vi "_PC_RTFunc_MSAnalExeCmd.vi"(5 "sv refnum":T1, 7 "Function":enum16{"Query", "Start", "Pause"}(ring)=enum."Start", 8 "error in (no error)":errorcluster, 9 "MS.Pause":refnum<vi>, 10 "MS.Start":refnum<vi>, 11 "Loops in":i32) -> (0 "error out":errorcluster, 1 "MSAnalExe?":bool, 2 "ExeTimes Out":i32)   [LabVIEW 2018]
uses:
  <vilib>/Utility/error.llb/Error Cluster From Error Code.vi
  <vilib>/ErrorRing/Error Ring.xnode
  <resource>/objmgr/ni.var.rc
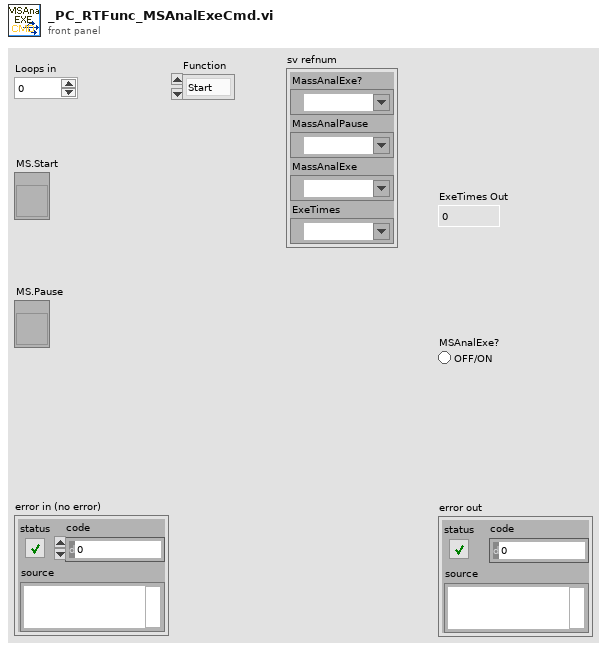
[diagram p1: front panel]
types:
  T1 = cluster{"MassAnalExe?":refnum<k21>, "MassAnalPause":refnum<k21>, "MassAnalExe":refnum<k21>, "ExeTimes":refnum<k21>}
  T2 = enum8{"Enabled", "Disabled", "Disabled and Grayed Out"}
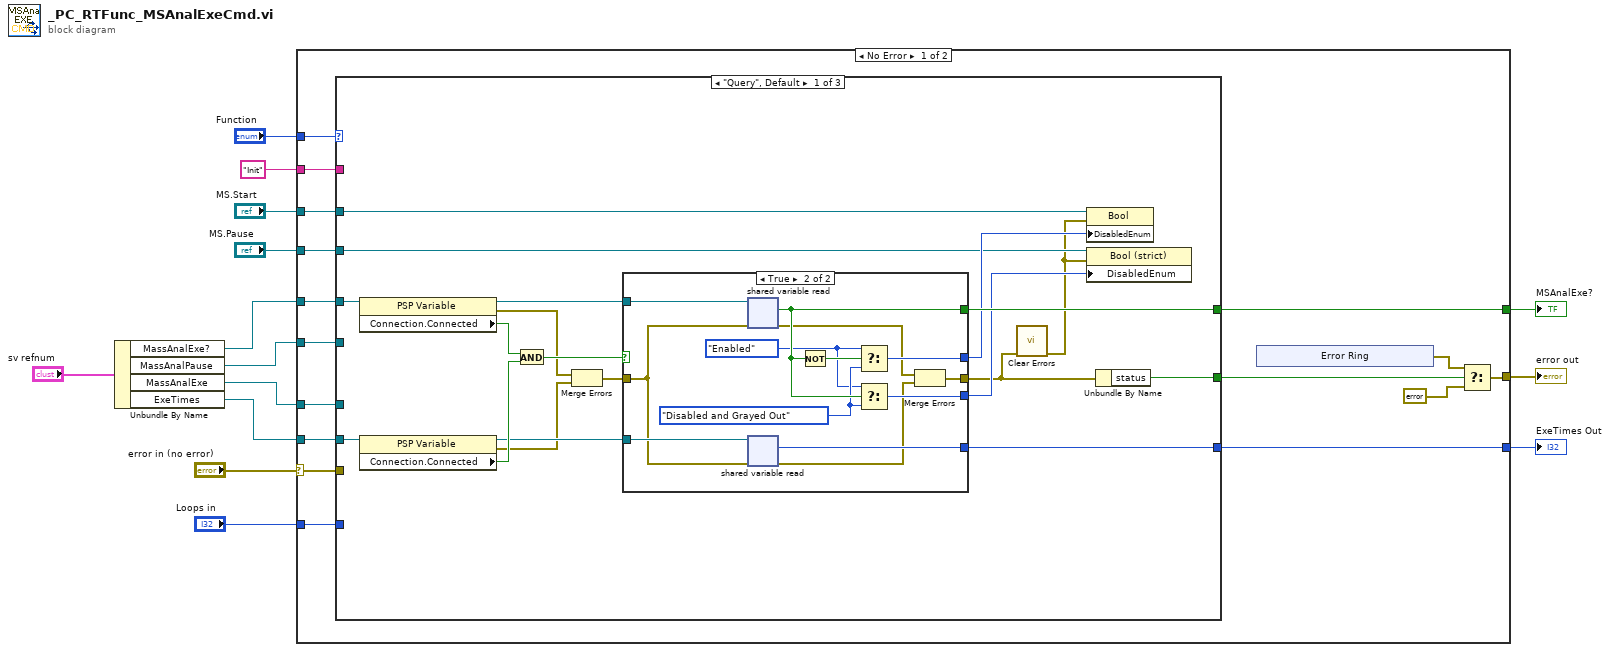
[diagram p0: block diagram]
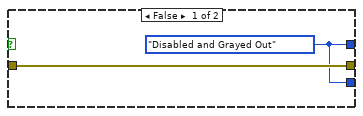
[diagram p2: hidden frame]
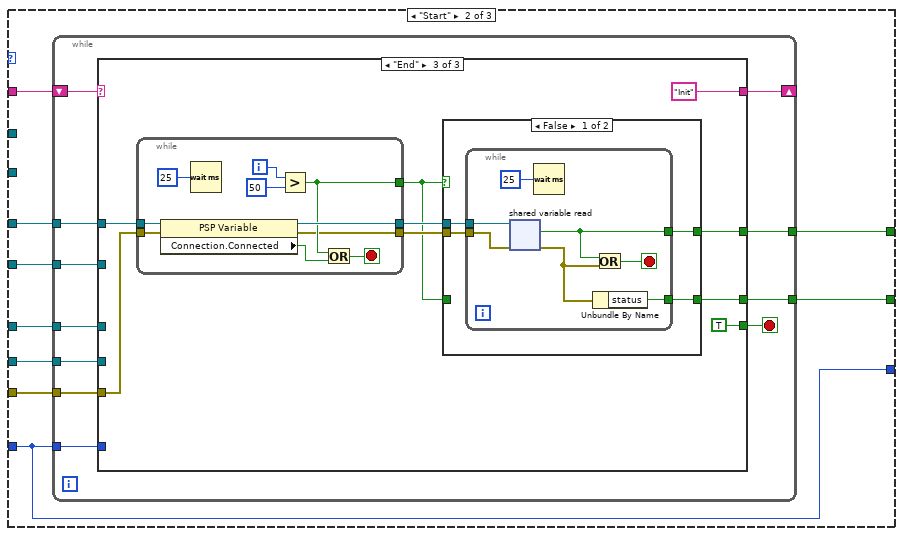
[diagram p3: hidden frame]
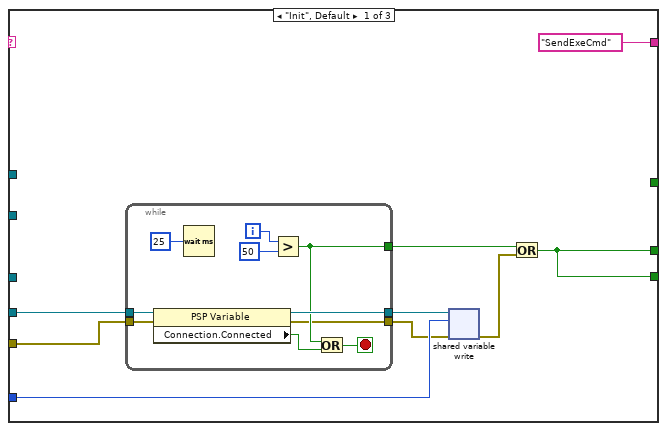
[diagram p4: hidden frame]
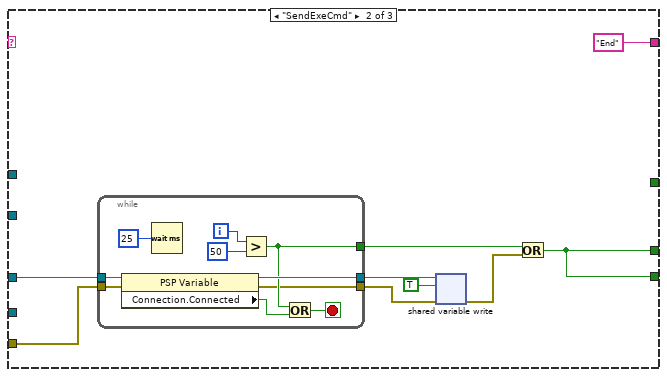
[diagram p5: hidden frame]
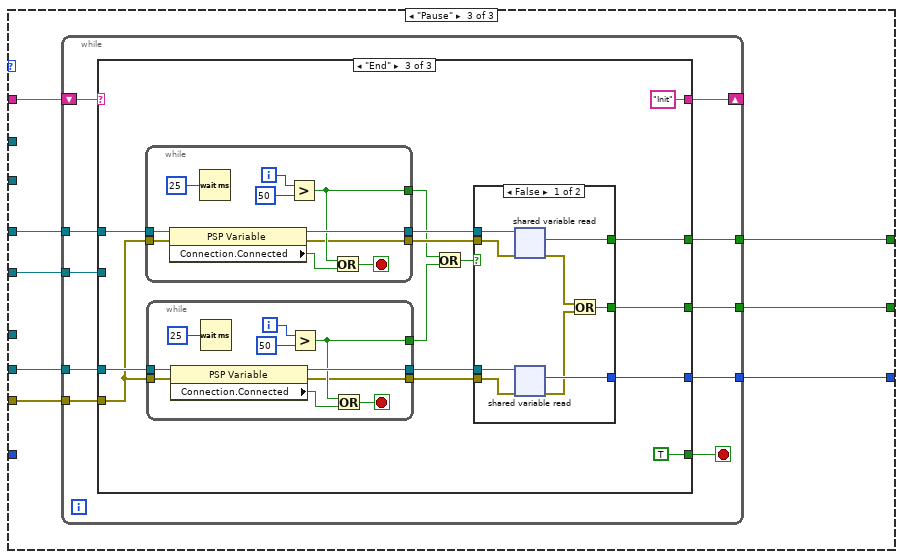
[diagram p7: hidden frame]
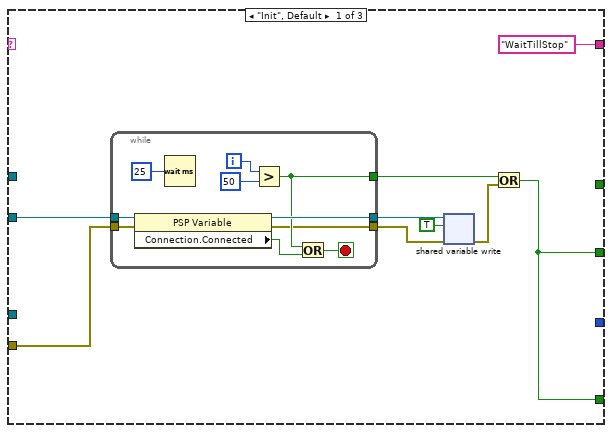
[diagram p8: hidden frame]
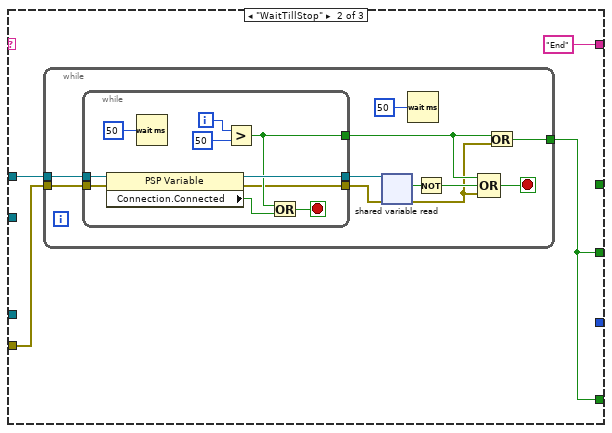
[diagram p9: hidden frame]
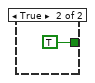
[diagram p10: hidden frame]
diagram:
  n1 = Unbundle By Name("sv refnum") -> ("MassAnalExe?"=w5:refnum<k21>, "MassAnalPause"=w4:refnum<k21>, "MassAnalExe"=w3:refnum<k21>, "ExeTimes"=w2:refnum<k21>)
  n2 = case shown="No Error" "error in (no error)" {
    selector: "error in (no error)" -> [w28 w265]
    tunnel: [w30 w265] -> w8
    tunnel: w5 -> [w20 _]
    tunnel: w4 -> [w19 _]
    tunnel: w3 -> [w18 _]
    tunnel: w2 -> [w17 _]
    tunnel: "Function" -> [w27 _]
    tunnel: "Init" -> [w23 _]
    tunnel: "MS.Start" -> [w24 _]
    tunnel: "MS.Pause" -> [w25 _]
    tunnel: "Loops in" -> [w26 _]
    tunnel: [w22 _] -> w10
    tunnel: [w21 _] -> w9
    frame No Error {
      n3 = case shown="\"Query\", Default" w27 {
        tunnel: w20 -> [w53 w72 w161]
        tunnel: w28 -> [_ w75 w163]
        tunnel: w19 -> [_ w73 w164]
        tunnel: w18 -> [_ w70 _]
        tunnel: w17 -> [w52 w76 w160]
        tunnel: [w47 w69 w158] -> w21
        tunnel: [w45 w71 w159] -> w22
        tunnel: w23 -> [_ w77 w165]
        tunnel: w26 -> [_ w69 _]
        tunnel: [w37 w74 w162] -> w16
        tunnel: w24 -> [w42 _ _]
        tunnel: w25 -> [w41 _ _]
        frame "Query", Default {
          n4 = property class="PSP Variable"(reference=w53) -> (reference out=w46:refnum<k21>, error out=w40:errorcluster, "Connection.Connected"=w51:bool)  [unwired: 1 in]
          n5 = property class="PSP Variable"(reference=w52) -> (reference out=w48:refnum<k21>, error out=w39:errorcluster, "Connection.Connected"=w50:bool)  [unwired: 1 in]
          n6 = And(x=w51, y=w50) -> (x .and. y?=w49:bool)
          n7 = Merge Errors(w40, w39) -> (w38:errorcluster)
          n8 = case shown="True" w49 {
            tunnel: w48 -> [_ w68]
            tunnel: [_ w67] -> w47
            tunnel: w46 -> [_ w66]
            tunnel: [_ w64] -> w45
            tunnel: [w54 w61] -> w44
            tunnel: [w54 w60] -> w43
            tunnel: [w55 w56] -> w36
            tunnel: w38 -> [w55 w59]
            frame False {
              w54 = T2."Disabled and Grayed Out" ("Disabled")
            }
            frame True {
              w62 = T2."Enabled" ("Disabled")
              w63 = T2."Disabled and Grayed Out" ("Disabled")
              n9 = shared-variable-read(w66, w59) -> (w58:errorcluster, w64:bool)  [unwired: 1 out]
              n10 = shared-variable-read(w68, w59) -> (w57:errorcluster, w67:i32)  [unwired: 1 out]
              n11 = Not(x=w64) -> (.not. x?=w65:bool)
              n12 = Select(t=w62, s=w65, f=w63) -> (s? t:f=w61:T2)
              n13 = Select(t=w62, s=w64, f=w63) -> (s? t:f=w60:T2)
              n14 = Merge Errors(w58, w57) -> (w56:errorcluster)
            }
          }
          n15 = call <vilib>:"Clear Errors.vi"("error in (no error)"=w36) -> ("error out"=w35:errorcluster)  [unwired: 5 in, 1 out]
          n16 = property class="Bool"(reference=w42, error in=w35, "DisabledEnum"=w44) -> ()  [unwired: 2 out]
          n17 = property class="Bool (strict)"(reference=w41, error in=w35, "DisabledEnum"=w43) -> ()  [unwired: 2 out]
          n18 = Unbundle By Name(w36) -> ("status"=w37:bool)
        }
        frame "Start" {
          n19 = while {
            shift-right: [w87] -> _
            shift-left: w77 -> [w88]
            tunnel: w76 -> [w86]
            tunnel: w75 -> [w85]
            tunnel: w69 -> [w84]
            tunnel: w73 -> [w82]
            tunnel: w72 -> [w81]
            tunnel: [w79] -> w71
            tunnel: w70 -> [w78]
            tunnel: [w83] -> w74
            stop <- w80 stop-if-true
            n20 = case shown="\"End\"" w88 {
              tunnel: ["SendExeCmd" "End" "Init"] -> w87
              tunnel: w86 -> [w97 _ _]
              tunnel: w85 -> [w96 w112 w134]
              tunnel: w84 -> [w94 _ _]
              tunnel: [w89 w108 w133] -> w83
              tunnel: w82 -> [_ _ _]
              tunnel: w81 -> [_ _ w135]
              tunnel: [w89 w108 TRUE] -> w80
              tunnel: [_ _ w132] -> w79
              tunnel: w78 -> [_ w113 _]
              frame "Init", Default {
                n21 = while {
                  tunnel: w97 -> [w107]
                  tunnel: w96 -> [w106]
                  tunnel: [w105] -> w95
                  tunnel: [w99] -> w92
                  tunnel: [w98] -> w93
                  i -> [w102]
                  stop <- w100 stop-if-true
                  n22 = property class="PSP Variable"(reference=w107, error in=w106) -> (reference out=w105:refnum<k21>, error out=w98:errorcluster, "Connection.Connected"=w101:bool)
                  n23 = Wait (ms)(milliseconds to wait=u32 25) -> ()  [unwired: 1 out]
                  n24 = Greater?(x=w102, y=50) -> (0:w99:bool)
                  n25 = Or(x=w99, y=w101) -> (x .or. y?=w100:bool)
                }
                n26 = shared-variable-write(w95, w93, w94) -> (w91:errorcluster)  [unwired: 1 out]
                n27 = Or(x=w92, y=w91) -> (x .or. y?=w89:bool)
              }
              frame "SendExeCmd" {
                n28 = while {
                  tunnel: w113 -> [w126]
                  tunnel: w112 -> [w125]
                  tunnel: [w124] -> w116
                  tunnel: [w118] -> w109
                  tunnel: [w117] -> w115
                  i -> [w121]
                  stop <- w119 stop-if-true
                  n29 = property class="PSP Variable"(reference=w126, error in=w125) -> (reference out=w124:refnum<k21>, error out=w117:errorcluster, "Connection.Connected"=w120:bool)
                  n30 = Wait (ms)(milliseconds to wait=u32 25) -> ()  [unwired: 1 out]
                  n31 = Greater?(x=w121, y=50) -> (0:w118:bool)
                  n32 = Or(x=w118, y=w120) -> (x .or. y?=w119:bool)
                }
                n33 = shared-variable-write(w116, w115, TRUE ("data in")) -> (w110:errorcluster)  [unwired: 1 out]
                n34 = Or(x=w109, y=w110) -> (x .or. y?=w108:bool)
              }
              frame "End" {
                n35 = while {
                  tunnel: w135 -> [w157]
                  tunnel: w134 -> [w156]
                  tunnel: [w155] -> w130
                  tunnel: [w149] -> w128
                  tunnel: [w148] -> w129
                  i -> [w152]
                  stop <- w150 stop-if-true
                  n36 = property class="PSP Variable"(reference=w157, error in=w156) -> (reference out=w155:refnum<k21>, error out=w148:errorcluster, "Connection.Connected"=w151:bool)
                  n37 = Wait (ms)(milliseconds to wait=u32 25) -> ()  [unwired: 1 out]
                  n38 = Greater?(x=w152, y=50) -> (0:w149:bool)
                  n39 = Or(x=w149, y=w151) -> (x .or. y?=w150:bool)
                }
                n40 = case shown="False" w128 {
                  tunnel: [w136 w147] -> w133
                  tunnel: [w139 _] -> w132
                  tunnel: w130 -> [w138 _]
                  tunnel: w129 -> [w137 _]
                  tunnel: w128 -> [_ w147]
                  frame False {
                    n41 = while {
                      tunnel: [w143] -> w139
                      tunnel: w138 -> [w146]
                      tunnel: w137 -> [w145]
                      tunnel: [w140] -> w136
                      stop <- w142 stop-if-true
                      n42 = shared-variable-read(w146, w145) -> (w141:errorcluster, w143:bool)  [unwired: 1 out]
                      n43 = Wait (ms)(milliseconds to wait=u32 25) -> ()  [unwired: 1 out]
                      n44 = Unbundle By Name(w141) -> ("status"=w140:bool)
                      n45 = Or(x=w143, y=w141) -> (x .or. y?=w142:bool)
                    }
                  }
                  frame True {
                  }
                }
              }
            }
          }
        }
        frame "Pause" {
          n46 = while {
            shift-right: [w172] -> _
            shift-left: w165 -> [w171]
            tunnel: w164 -> [w175]
            tunnel: w163 -> [w174]
            tunnel: [w173] -> w162
            tunnel: w161 -> [w170]
            tunnel: w160 -> [w169]
            tunnel: [w168] -> w159
            tunnel: [w167] -> w158
            stop <- w166 stop-if-true
            n47 = case shown="\"End\"" w171 {
              tunnel: w175 -> [w184 _ _]
              tunnel: w174 -> [w183 w197 w232]
              tunnel: [w177 w195 w222] -> w173
              tunnel: ["WaitTillStop" "End" ("t") "Init" ("t")] -> w172
              tunnel: w170 -> [_ w196 w234]
              tunnel: w169 -> [_ _ w233]
              tunnel: [_ _ w227] -> w168
              tunnel: [_ _ w226] -> w167
              tunnel: [w177 w195 TRUE] -> w166
              frame "Init", Default {
                n48 = while {
                  tunnel: w184 -> [w194]
                  tunnel: w183 -> [w193]
                  tunnel: [w192] -> w182
                  tunnel: [w186] -> w178
                  tunnel: [w185] -> w181
                  i -> [w189]
                  stop <- w187 stop-if-true
                  n49 = property class="PSP Variable"(reference=w194, error in=w193) -> (reference out=w192:refnum<k21>, error out=w185:errorcluster, "Connection.Connected"=w188:bool)
                  n50 = Wait (ms)(milliseconds to wait=u32 25) -> ()  [unwired: 1 out]
                  n51 = Greater?(x=w189, y=50) -> (0:w186:bool)
                  n52 = Or(x=w186, y=w188) -> (x .or. y?=w187:bool)
                }
                n53 = shared-variable-write(w182, w181, TRUE ("data in")) -> (w179:errorcluster)  [unwired: 1 out]
                n54 = Or(x=w178, y=w179) -> (x .or. y?=w177:bool)
              }
              frame "WaitTillStop" {
                n55 = while {
                  tunnel: w197 -> [w209]
                  tunnel: w196 -> [w208]
                  tunnel: [w199] -> w195
                  stop <- w202 stop-if-true
                  n56 = while {
                    tunnel: w208 -> [w219]
                    tunnel: w209 -> [w218]
                    tunnel: [w217] -> w207
                    tunnel: [w211] -> w201
                    tunnel: [w210] -> w206
                    i -> [w214]
                    stop <- w212 stop-if-true
                    n57 = property class="PSP Variable"(reference=w219, error in=w218) -> (reference out=w217:refnum<k21>, error out=w210:errorcluster, "Connection.Connected"=w213:bool)
                    n58 = Wait (ms)(milliseconds to wait=u32 50) -> ()  [unwired: 1 out]
                    n59 = Greater?(x=w214, y=50) -> (0:w211:bool)
                    n60 = Or(x=w211, y=w213) -> (x .or. y?=w212:bool)
                  }
                  n61 = shared-variable-read(w207, w206) -> (w200:errorcluster, w204:bool)  [unwired: 1 out]
                  n62 = Wait (ms)(milliseconds to wait=u32 50) -> ()  [unwired: 1 out]
                  n63 = Not(x=w204) -> (.not. x?=w203:bool)
                  n64 = Compound Arithmetic op=OR(w201, w203, w200) -> (w202:bool)
                  n65 = Or(x=w201, y=w200) -> (x .or. y?=w199:bool)
                }
              }
              frame "End" {
                n66 = while {
                  tunnel: w234 -> [w264]
                  tunnel: w232 -> [w263]
                  tunnel: [w262] -> w231
                  tunnel: [w256] -> w224
                  tunnel: [w255] -> w230
                  i -> [w259]
                  stop <- w257 stop-if-true
                  n67 = property class="PSP Variable"(reference=w264, error in=w263) -> (reference out=w262:refnum<k21>, error out=w255:errorcluster, "Connection.Connected"=w258:bool)
                  n68 = Wait (ms)(milliseconds to wait=u32 25) -> ()  [unwired: 1 out]
                  n69 = Greater?(x=w259, y=50) -> (0:w256:bool)
                  n70 = Or(x=w256, y=w258) -> (x .or. y?=w257:bool)
                }
                n71 = while {
                  tunnel: w233 -> [w254]
                  tunnel: w232 -> [w253]
                  tunnel: [w252] -> w229
                  tunnel: [w246] -> w223
                  tunnel: [w245] -> w228
                  i -> [w249]
                  stop <- w247 stop-if-true
                  n72 = property class="PSP Variable"(reference=w254, error in=w253) -> (reference out=w252:refnum<k21>, error out=w245:errorcluster, "Connection.Connected"=w248:bool)
                  n73 = Wait (ms)(milliseconds to wait=u32 25) -> ()  [unwired: 1 out]
                  n74 = Greater?(x=w249, y=50) -> (0:w246:bool)
                  n75 = Or(x=w246, y=w248) -> (x .or. y?=w247:bool)
                }
                n76 = Or(x=w224, y=w223) -> (x .or. y?=w225:bool)
                n77 = case shown="False" w225 {
                  tunnel: w231 -> [w243 _]
                  tunnel: w230 -> [w242 _]
                  tunnel: w229 -> [w241 _]
                  tunnel: w228 -> [w240 _]
                  tunnel: [w239 _] -> w227
                  tunnel: [w238 _] -> w226
                  tunnel: [w235 TRUE] -> w222
                  frame False {
                    n78 = shared-variable-read(w243, w242) -> (w237:errorcluster, w239:bool)  [unwired: 1 out]
                    n79 = shared-variable-read(w241, w240) -> (w236:errorcluster, w238:i32)  [unwired: 1 out]
                    n80 = Or(x=w237, y=w236) -> (x .or. y?=w235:bool)
                  }
                  frame True {
                  }
                }
              }
            }
          }
        }
      }
      n81 = xnode "Error Ring"() -> ("error out"=w15:errorcluster)
      n82 = Select(t=w15, s=w16, f=errorcluster {"status"=FALSE, "code"=0, "source"=""} ("error constant")) -> (s? t:f=w30:errorcluster)
    }
    frame Error {
    }
  }
  "error out" <- w8
  "MSAnalExe?" <- w10
  "ExeTimes Out" <- w9
